vi "Calculate_PID_Discrete_Coeff(SubVI).vi"(10 "PID_in":T3, 11 "Controller type":T1) -> (2 "PID_Discrete_Out":T2)   [LabVIEW 2017]
uses:
  PID_Discrete_Coefficients.ctl
  Controller_Type.ctl
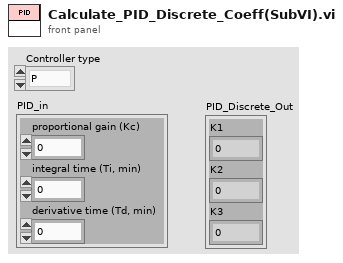
[diagram p1: front panel]
types:
  T1 = typedef "Controller_Type.ctl" = enum16{"P", "PI", "PD", "PID"}
  T2 = typedef "PID_Discrete_Coefficients.ctl" = cluster{"K1":dbl, "K2":dbl, "K3":dbl}
  T3 = cluster{"proportional gain (Kc)":dbl, "integral time (Ti, min)":dbl, "derivative time (Td, min)":dbl}
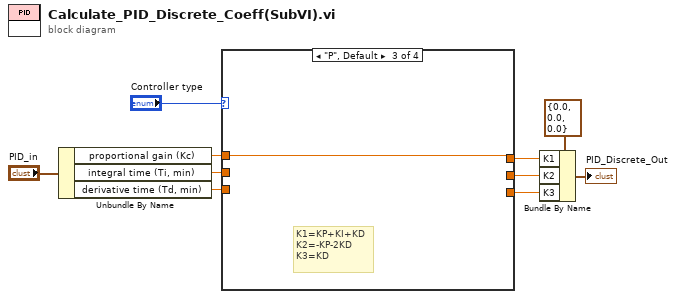
[diagram p0: block diagram]
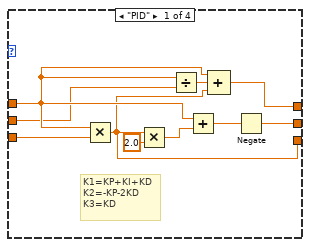
[diagram p2: hidden frame]
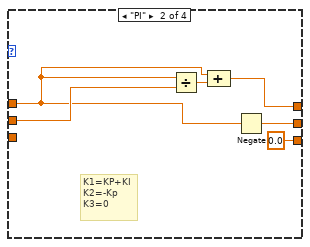
[diagram p3: hidden frame]
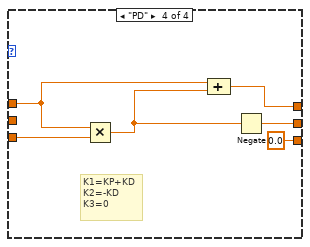
[diagram p4: hidden frame]
diagram:
  n1 = Unbundle By Name("PID_in") -> ("proportional gain (Kc)"=w10:dbl, "integral time (Ti, min)"=w8:dbl, "derivative time (Td, min)"=w9:dbl)
  n2 = case shown="\"P\", Default" "Controller type" {
    tunnel: w10 -> [w20 w22 w27 w30]
    tunnel: w9 -> [w19 _ _ w33]
    tunnel: w8 -> [w18 w26 _ _]
    tunnel: [w17 0.0 _ 0.0] -> w5
    tunnel: [w16 w25 _ w32] -> w4
    tunnel: [w12 w24 w27 w31] -> w3
    frame "PID" {
      # "K1=KP+KI+KD\nK2=-KP-2KD\nK3=KD"
      n3 = Multiply(x=w20, y=w19) -> (x*y=w17:dbl)
      n4 = Multiply(x=w17, y=2.0) -> (x*y=w14:dbl)
      n5 = Divide(x=w20, y=w18) -> (x/y=w11:dbl)
      n6 = Add(x=w20, y=w14) -> (x+y=w15:dbl)
      n7 = Compound Arithmetic op=ADD(w20, w11, w17) -> (w12:dbl)
      n8 = Negate(x=w15) -> (-x=w16:dbl)
    }
    frame "PI" {
      # "K1=KP+KI\nK2=-Kp\nK3=0"
      n9 = Divide(x=w22, y=w26) -> (x/y=w23:dbl)
      n10 = Compound Arithmetic op=ADD(w22, w23) -> (w24:dbl)
      n11 = Negate(x=w22) -> (-x=w25:dbl)
    }
    frame "P", Default {
      # "K1=KP+KI+KD\nK2=-KP-2KD\nK3=KD"
    }
    frame "PD" {
      # "K1=KP+KD\nK2=-KD\nK3=0"
      n12 = Multiply(x=w30, y=w33) -> (x*y=w28:dbl)
      n13 = Compound Arithmetic op=ADD(w30, w28) -> (w31:dbl)
      n14 = Negate(x=w28) -> (-x=w32:dbl)
    }
  }
  n15 = Bundle By Name(cluster=T2 {"K1"=0.0, "K2"=0.0, "K3"=0.0} ("PID DISCRETE"), "K1"=w3, "K2"=w4, "K3"=w5) -> (→"PID_Discrete_Out":T2)
